vi "FTW-Connector-Tell.vi"(0 "FTW Actor Connector":refnum<class "FTW-ActorConnector.lvclass">, 5 "Message Header":string, 7 "Message Body":string, 9 "Timeout":i32=100 format="%dmsec", 11 "error in":errorcluster) -> (4 "FTW Actor Connector out":refnum<class "FTW-ActorConnector.lvclass">, 6 "Timed out?":bool, 15 "error out":errorcluster)   [LabVIEW 2013, in "FTW-ActorConnector.lvclass"]
uses:
  FTW-ActorConnector.lvclass
  FTW-ActorConnector.lvclass/FTW-ActorConnector.ctl
  Client/FTW-Client.lvclass
panel:
  # "Inputs"
  # "Outputs"
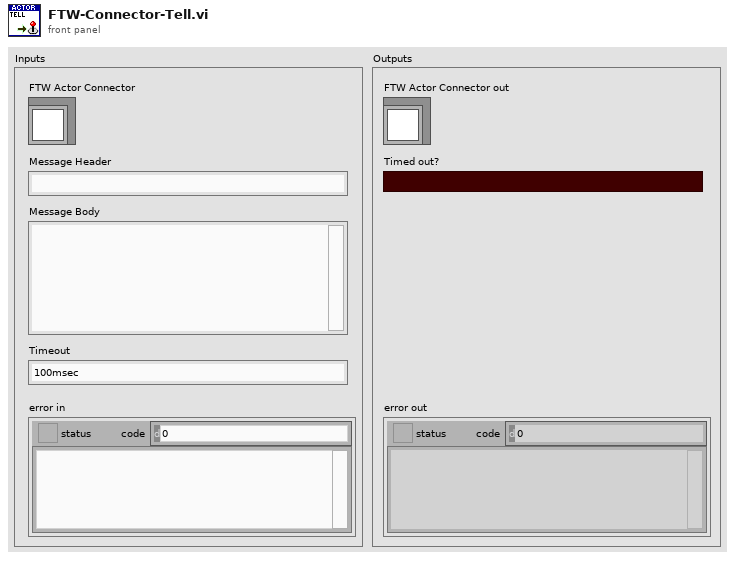
[diagram p1: front panel]
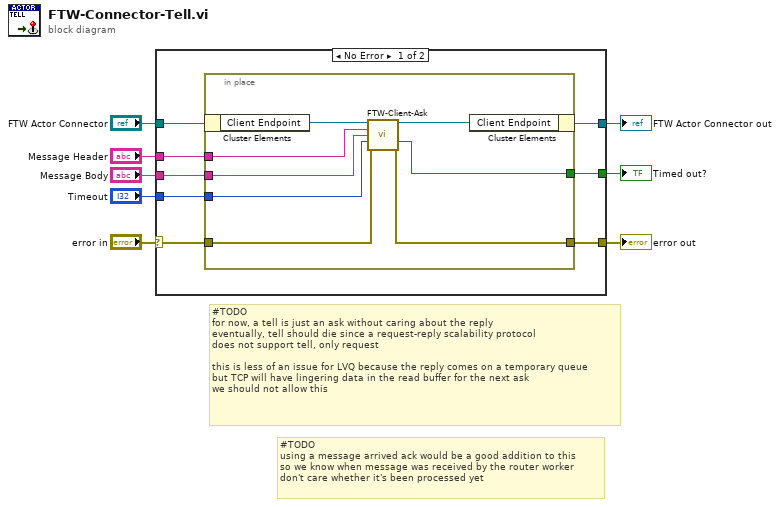
[diagram p0: block diagram]
diagram:
  # "#TODO\nusing a message arrived ack would be a good addition to this\nso we know when message was received by the router worker\ndon't care whether it's been processed yet"
  # "#TODO\nfor now, a tell is just an ask without caring about the reply\neventually, tell should die since a request-reply scalability protocol\ndoes not support tell, only request\n\nthis is less of an issue for LVQ because the reply comes on a temporary queue\nbut TCP will have lingering data in the read buffer for the next ask\nwe should not allow this"
  n1 = case shown="No Error" "error in" {
    selector: "error in" -> [w15 w26]
    tunnel: [w13 w26] -> w7
    tunnel: "FTW Actor Connector" -> [w16 w25]
    tunnel: [w14 w25] -> w5
    tunnel: "Message Header" -> [w12 _]
    tunnel: "Message Body" -> [w11 _]
    tunnel: "Timeout" -> [w10 _]
    tunnel: [w9 _] -> w1
    frame No Error {
      n2 = in-place {
        in-place-border: w15 -> [w24]
        in-place-border: [w23] -> w13
        in-place-border: w12 -> [w20]
        in-place-border: w11 -> [w19]
        in-place-border: w10 -> [w18]
        in-place-border: [w17] -> w9
        n3 = in-place-cluster #1(w16) -> ("Client Endpoint"=w22:refnum<class "FTW-Client.lvclass">)
        n4 = call "FTW-Client-Ask.vi"("FTW-Client In"=w22, "Header"=w20, "Body"=w19, "Timeout"=w18, "error in"=w24) -> ("FTW-Client Out"=w21:refnum<class "FTW-Client.lvclass">, "Timed out?"=w17:bool, "error out"=w23:errorcluster)  [unwired: 5 in, 3 out]
        n5 = in-place-cluster #1("Client Endpoint"=w21) -> (w14:refnum<class "FTW-ActorConnector.lvclass">)
      }
    }
    frame Error {
    }
  }
  "error out" <- w7
  "FTW Actor Connector out" <- w5
  "Timed out?" <- w1
